vi "Main 2.vi"() -> ()   [LabVIEW 2016, in "MyHostCode.lvlib"]
doc: "This VI was generated automatically using the FPGA Wizard. You can modify the VI normally."
uses:
  MyHostCode.lvlib
  FPGACode/Lead Enum.ctl
  Trigger Params.ctl
  FPGACode/Channel Enum.ctl
  <vilib>/Utility/file.llb/Write To Spreadsheet File (I64).vi
  <vilib>/FPGAPlugInAG/USB-7856R OEM/niLvFpga_Open_USB-7856R OEM.vi
  <vilib>/rvi/interface/common/dynamic/niFpgaDynamicAddResources.vi
  <vilib>/FPGAPlugInAG/Dynamic/niLvFpga_Reset_Dynamic.vi
  <vilib>/FPGAPlugInAG/Dynamic/niLvFpga_Run_Dynamic.vi
  <vilib>/Utility/error.llb/Error Cluster From Error Code.vi
  <vilib>/rvi/errors/niLvFpgaAdjustHostInterfaceError.vi
  <vilib>/FPGAPlugInAG/Dynamic/niLvFpga_Close_Dynamic.vi
  <vilib>/rvi/interface/nirviOpenFPGA/nirviOpenFPGA.xnode
  FPGA Bitfiles/ECGPWMAdaptiveFi_FPGATarget3_ECGAFSPIInput2_KN+BrzZOq5c.lvbitx
  <vilib>/rvi/interface/nirviMethod/nirviMethod.xnode
  <vilib>/rvi/interface/nirviReadWriteControl/nirviReadWriteControl.xnode
  <vilib>/rvi/interface/nirviCloseFPGA/nirviCloseFPGA.xnode
  <vilib>/rvi/interface/Simulation/niFpgaSimulationCallBeginRW.vi
  <vilib>/FPGAPlugInAG/Dynamic/niLvFpga_ReadFifo_Dynamic.vi
  <vilib>/rvi/errors/niLvFpgaMergeErrorWithErrorCode.vi
  NiFpgaLv.dll
panel:
  in  "Path":path=path "C:/Users/IFEUser/Documents/LabVIEW Data/Saved Data/test.txt"
  in  "Record":bool
  in  "Beta":u8(slide)=1 scale=0.0..3.0
  in  "Sensis\nECG Scaling":i16=1 caption="ECG Output\nScaling" min=1 max=100 step=1
  in  "Tab Control":enum32{"Main", "Utilities"}(tab)
  in  "IBP2":T1={"Scale"=0.169921875, "Offset"=-1935.0} {"Scale" format="%#_3g"}
  out "ECG":i16[][](graph)
  out "Invasive Blood Pressure":i16[][](graph)=[[-20, 4166], [-20, 4166], [-20, 4165], [-20, 4165], [-19, 4165], [-19, 4165], [-18, 4163], [-18, 4165], [-18, 4166], [-18, 4166], [-18, 4166], [-18, 4165], [-18, 4165], [-18, 4164], [-18, 4164], [-18, 4165], [-19, 4166], [-20, 4166], [-20, 4164], [-20, 4164], [-20, 4165], [-20, 4165], [-19, 4165], [-19, 4164], [-18, 4165], [-18, 4166], [-18, 4165], [-18, 4166], [-18, 4165], [-18, 4165], [-18, 4165], [-18, 4165], [-19, 4165], [-20, 4165], [-20, 4165], [-20, 4165], [-20, 4166], [-20, 4167], [-20, 4166], [-19, 4164], [-18, 4163], [-18, 4164], [-18, 4165], [-18, 4166], [-17, 4165], [-18, 4166], [-18, 4166], [-18, 4165], [-18, 4166], [-19, 4165], [-20, 4164], [-20, 4165], [-20, 4166], [-20, 4166], [-20, 4167]]
  in  "Trigger 2":T2={"Channel"=enum."II", "Threshold"=1000, "d/dt"=FALSE, "Invert"=FALSE}
  out "Trigger":i16[][](graph)
  in  "IBP Filter":bool
  in  "Plot Info":T5={"Element"={"Lead"=enum."I", "Filter"=TRUE}, "Element 2"={"Lead"=enum."II", "Filter"=TRUE}, "Element 3"={"Lead"=enum."III", "Filter"=TRUE}}
  in  "IBP1":T1={"Scale"=0.1669921875, "Offset"=-1795.0} {"Scale" format="%#_4g"}
  in  "Invert IBP PWM":bool=TRUE
  in  "Invert ECG PWM":bool=TRUE
  out "Gradients":i16[][](graph)
  in  "Offset":cluster{"X":i16, "Y":i16, "Z":i16} {"Z" format="%.2f"; "Y" format="%.2f"; "X" format="%.2f"}
  in  "High Pass Filter":bool
  out "Taps":dbl[](graph)
  out "Weights":dbl[](graph)
  out "Beta Product":fxp<+/-,32,-1> format="%.3e"
  out "Weighted Sum":fxp<+/-,33,19> format="%.3e"
  in  "Channel":i32
  in  "ECG Input\nGain":u16(ring)=1 items=["1"=1, "2"=2, "3"=3, "4"=4, "6"=0, "8"=5, "12"=6]
  in  "ECG Beta":fxp<+/-,32,-16>=1.000088900582341e-11 format="%.3e"
  in  "Filter Size":i16=100
  in  "IBP Beta":fxp<+/-,32,-16> format="%.3e"
  out "Loop Time":u32
  in  "Reset":bool
  out "Actual Loop Rate (Ticks)":u32
  out "Late? Latched":bool
  in  "Start":bool
  in  "Loop Rate (Hz)":dbl=10000.0
  out "Calculated Rate (Hz)":dbl
  out "error out":errorcluster
  in  "Global Stop":bool
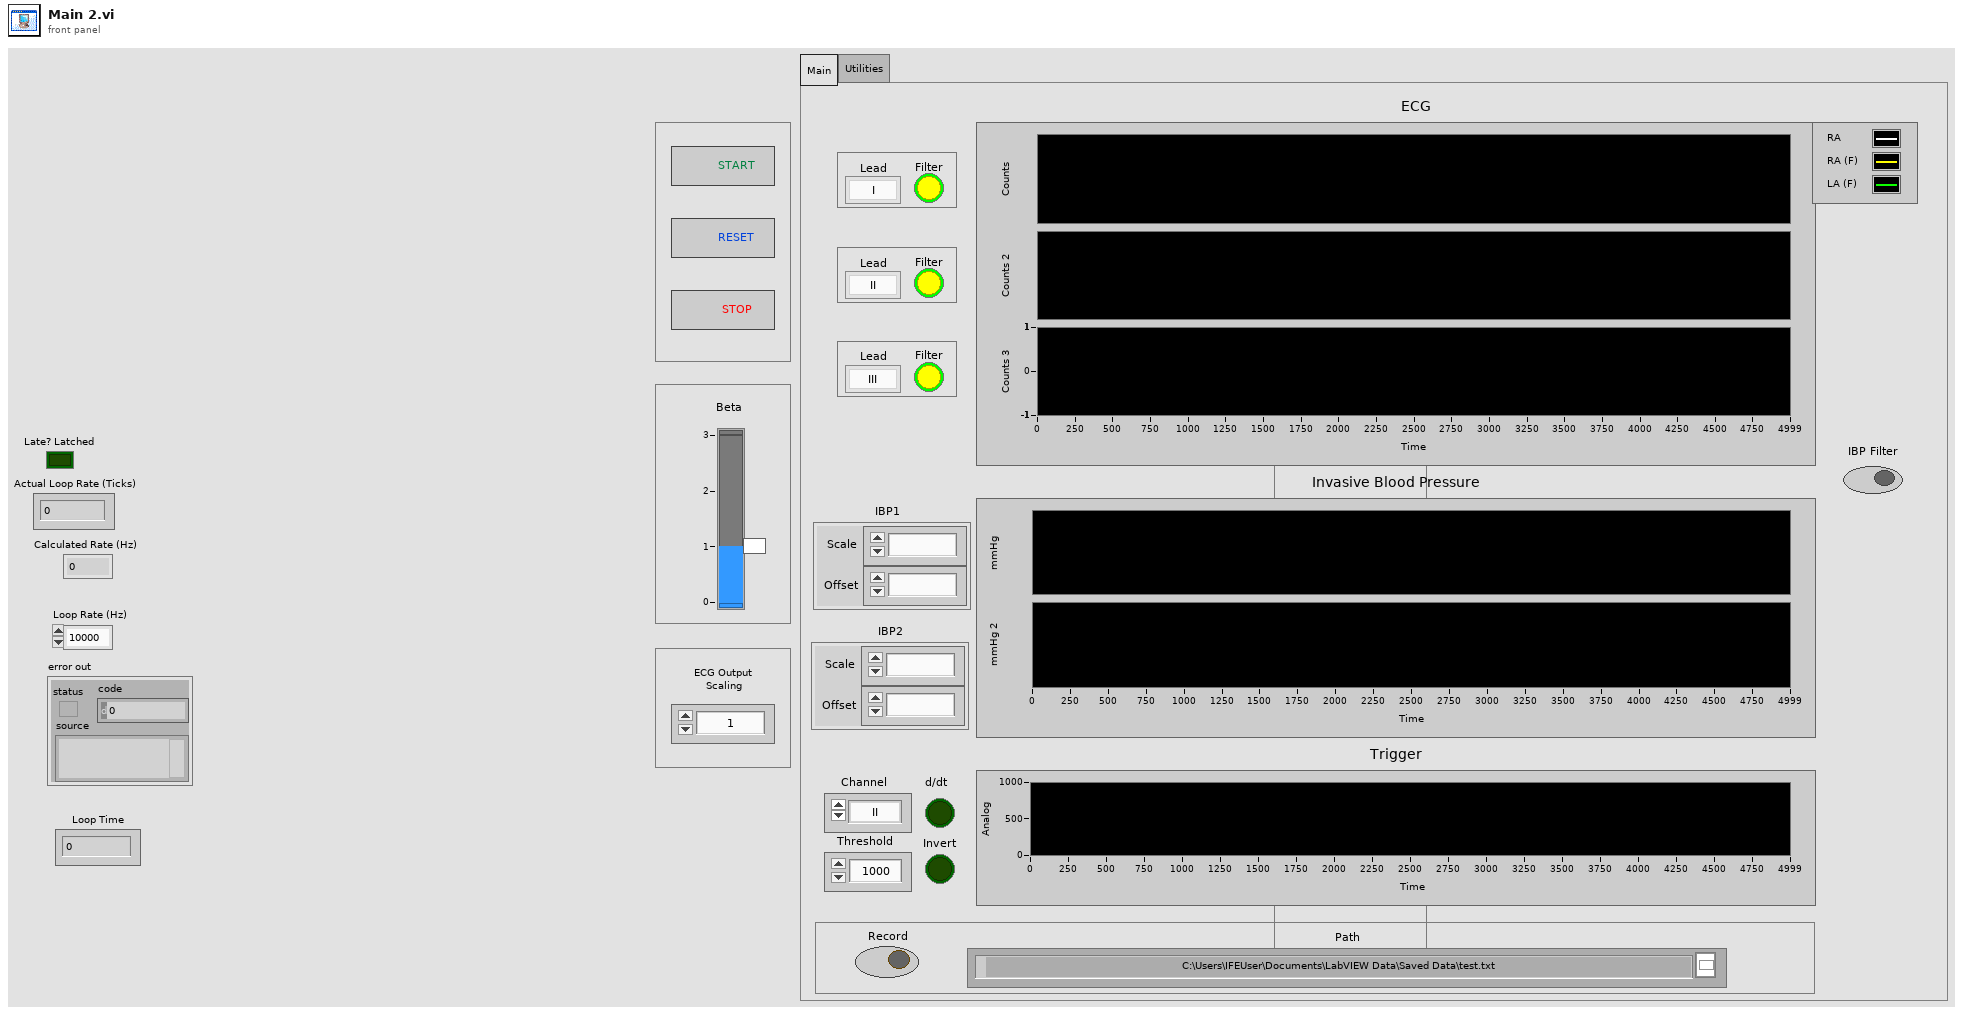
[diagram p1: front panel]
types:
  T1 = cluster{"Scale":fxp<+/-,16,5>, "Offset":fxp<+/-,16,16>}
  T2 = typedef "Trigger Params.ctl" = cluster{"Channel":T3, "Threshold":i16, "d/dt":bool, "Invert":bool}
  T3 = typedef "Channel Enum.ctl" = enum16{"RA", "LA", "LL", "V1", "V2", "V3", "V4", "V5", "V6", "I", "II", "III", "aVR", "aVL", "aVF", "Vw", "IBP1", "IBP2"}
  T4 = typedef "Lead Enum.ctl" = enum16{"RA", "LA", "LL", "V1", "V2", "V3", "V4", "V5", "V6", "I", "II", "III", "aVR", "aVL", "aVF", "Vw"}
  T5 = cluster{"Element":cluster{"Lead":T4, "Filter":bool}, "Element 2":cluster{"Lead":T4, "Filter":bool}, "Element 3":cluster{"Lead":T4, "Filter":bool}}
  T6 = enum8{"Enabled", "Disabled", "Disabled and Grayed Out"}
  T7 = typedef "LVOffsetAndMultiplierTypeDef.ctl" = cluster{"Offset":dbl, "Multiplier":dbl}
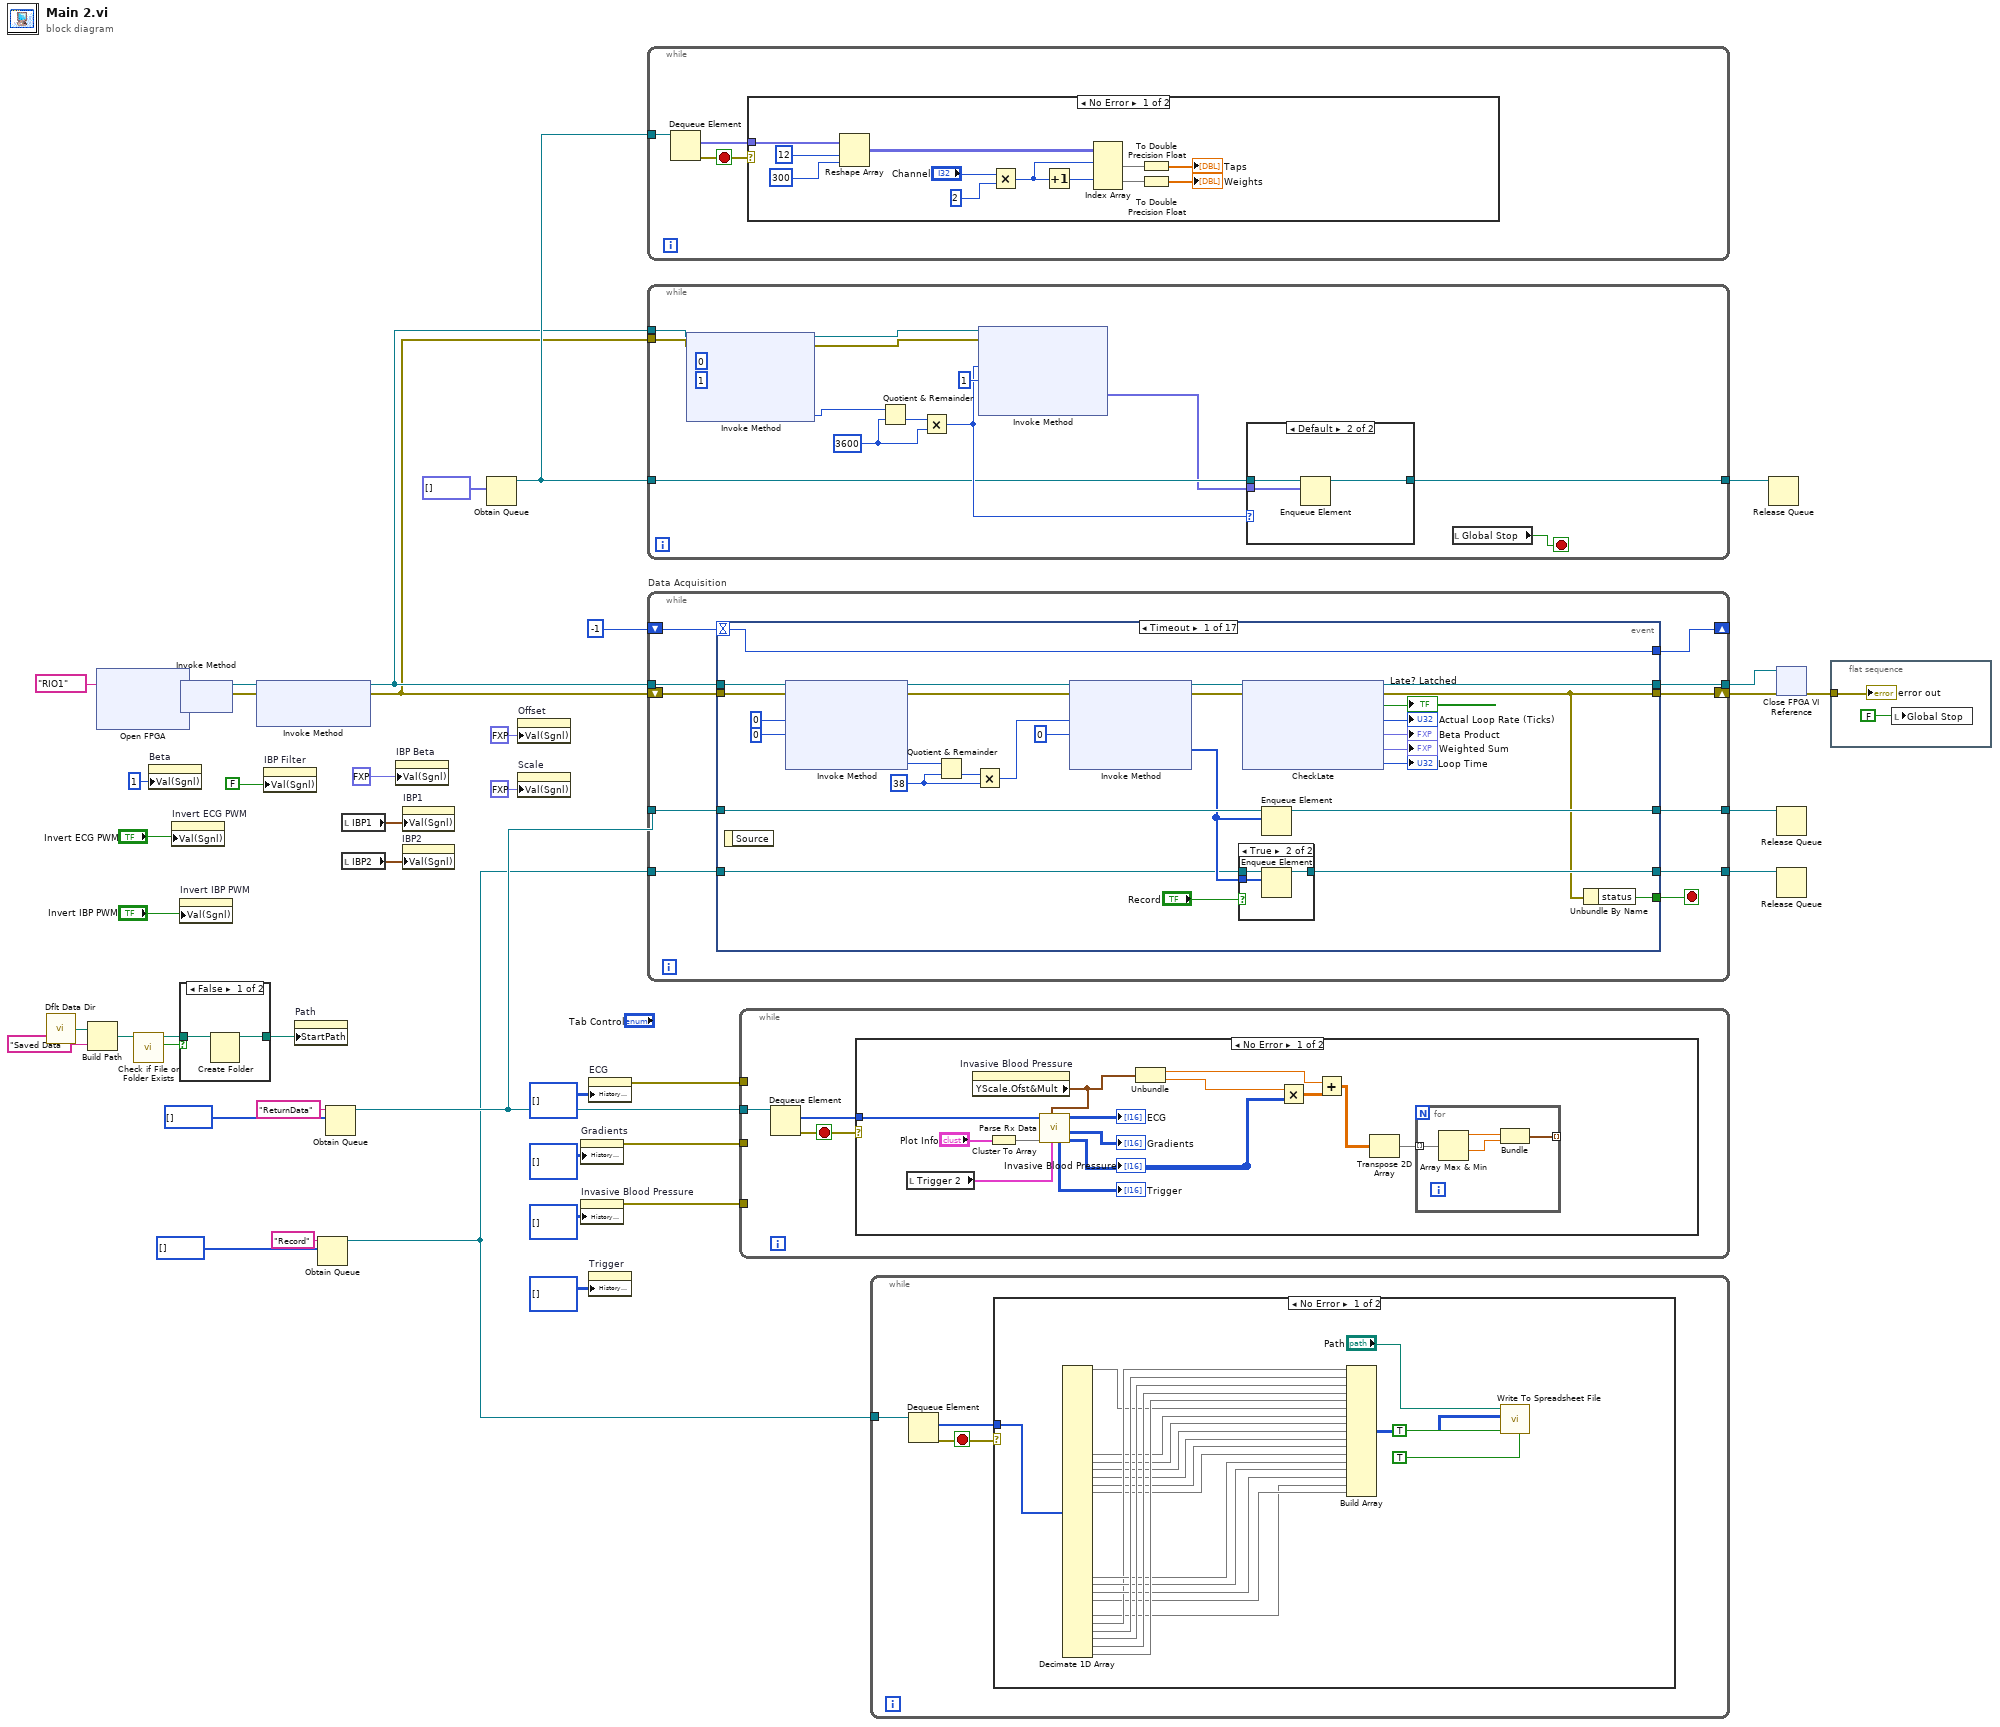
[diagram p0: block diagram]
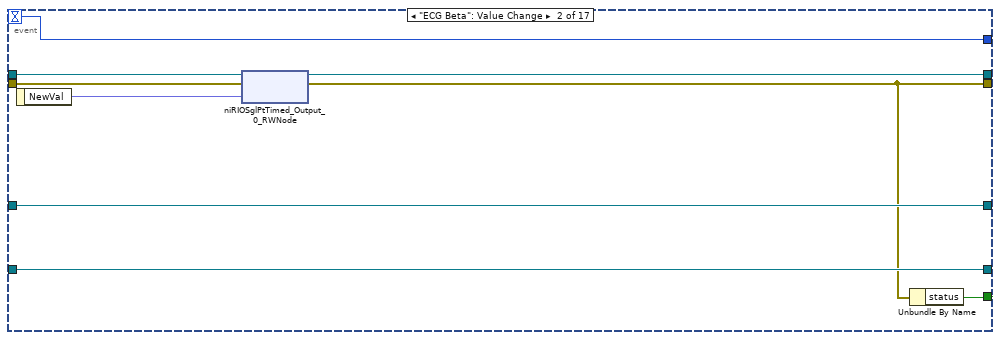
[diagram p4: hidden frame]
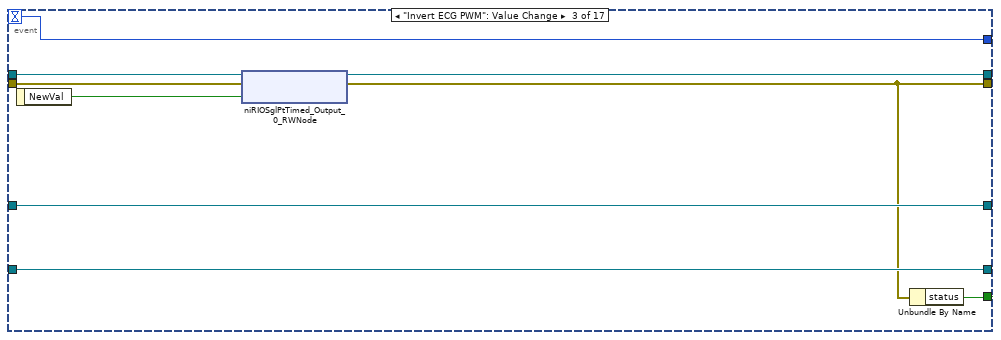
[diagram p5: hidden frame]
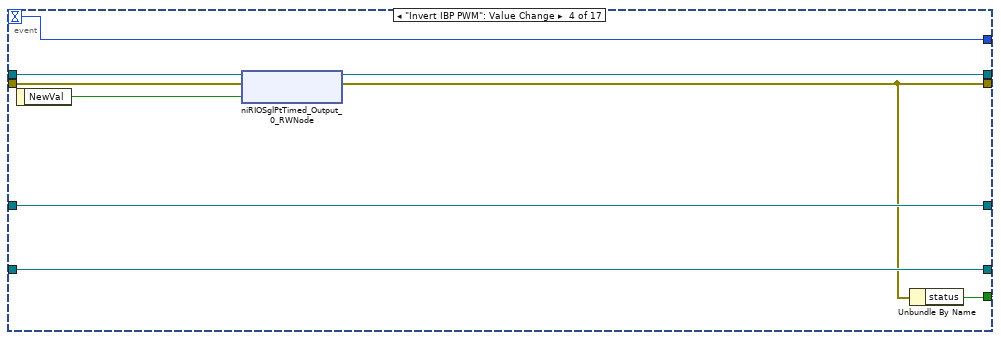
[diagram p6: hidden frame]
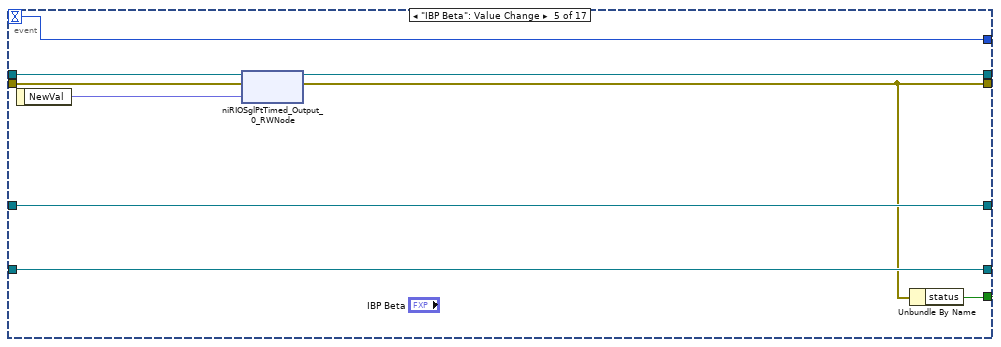
[diagram p7: hidden frame]
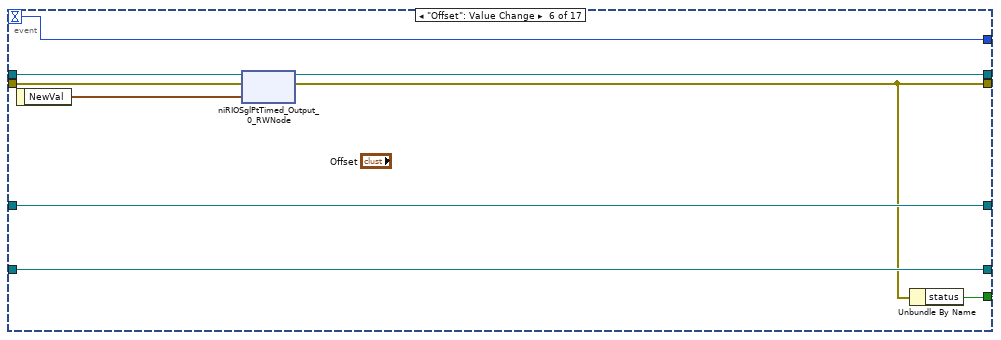
[diagram p8: hidden frame]
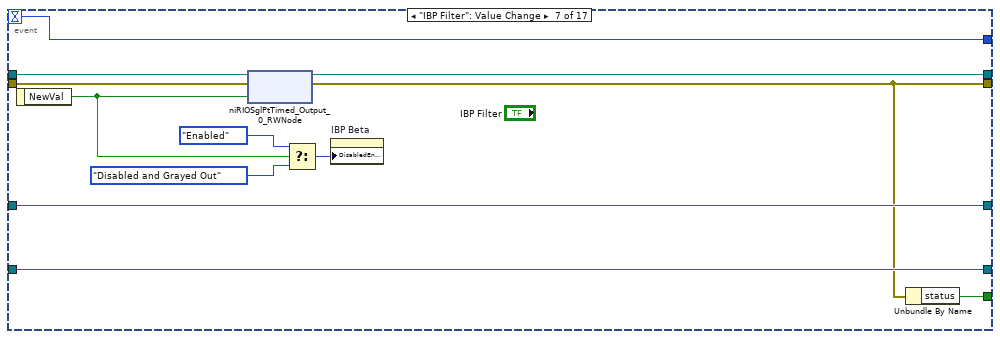
[diagram p9: hidden frame]
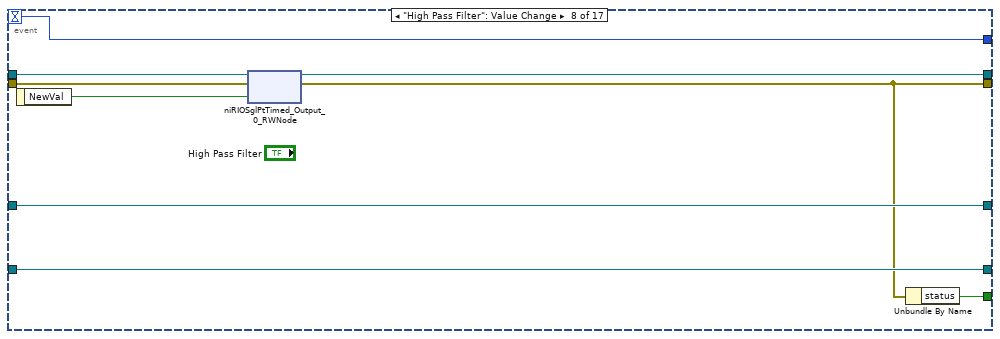
[diagram p10: hidden frame]
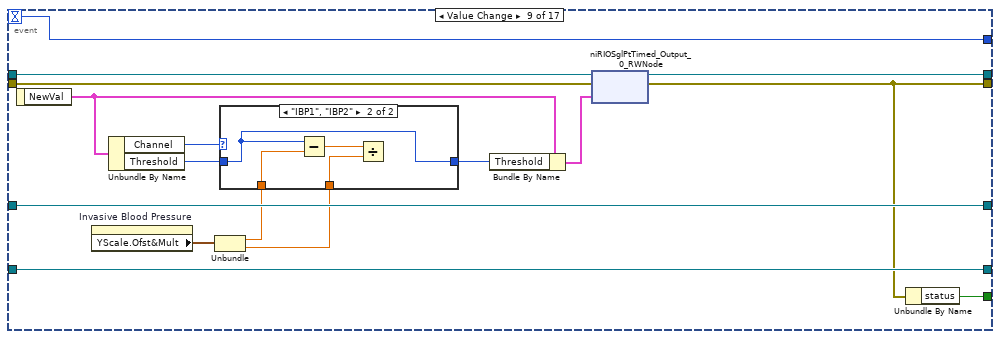
[diagram p11: hidden frame]
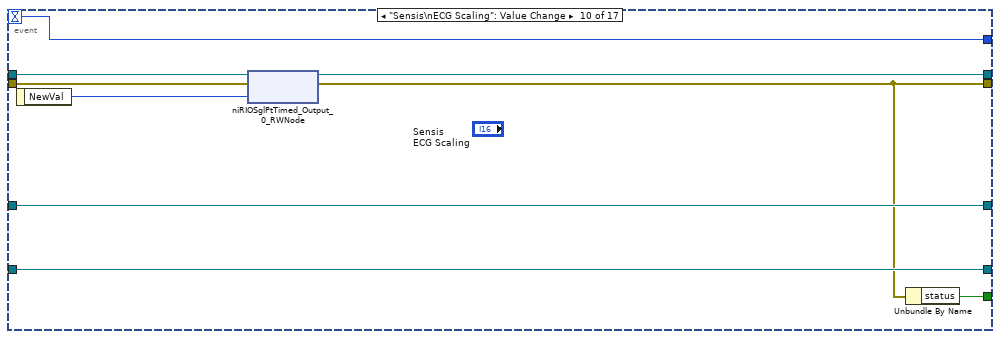
[diagram p13: hidden frame]
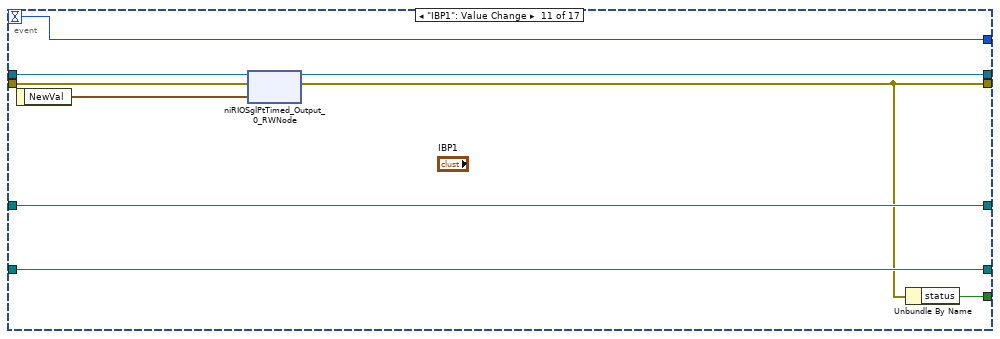
[diagram p14: hidden frame]
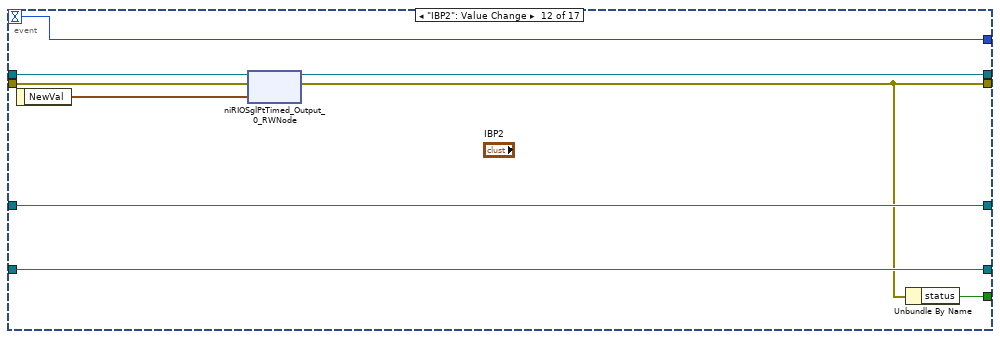
[diagram p15: hidden frame]
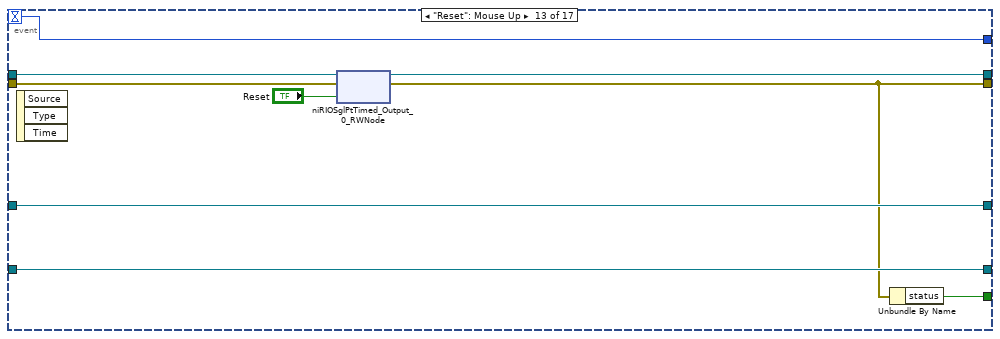
[diagram p16: hidden frame]
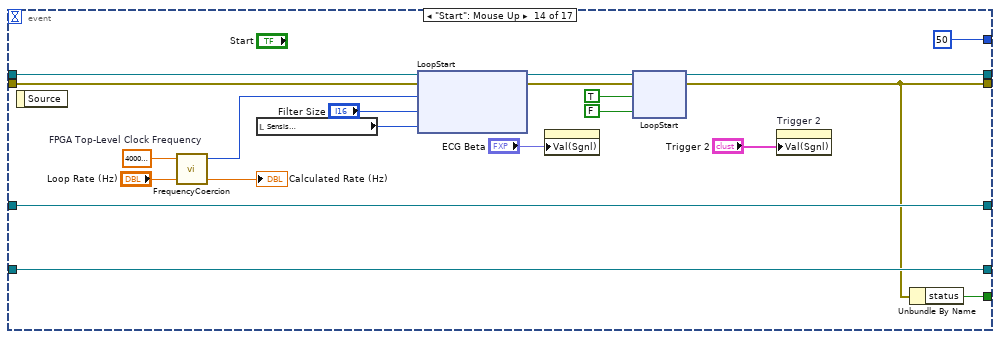
[diagram p17: hidden frame]
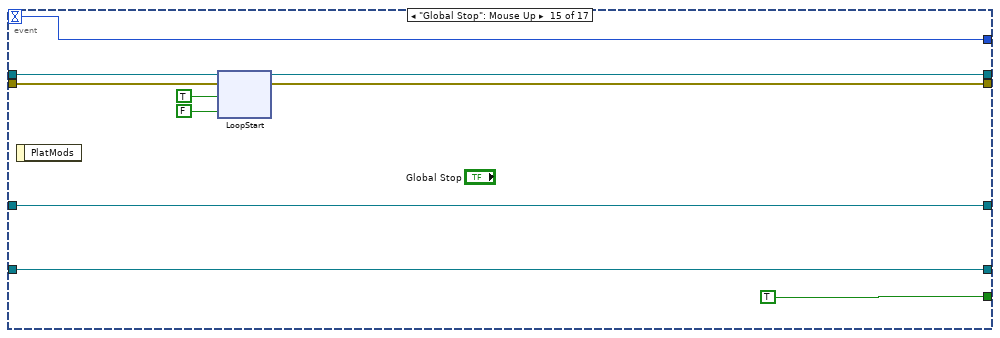
[diagram p18: hidden frame]
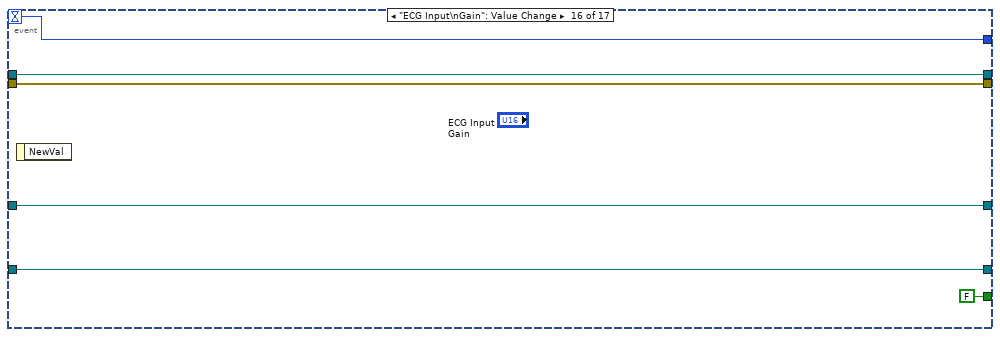
[diagram p19: hidden frame]
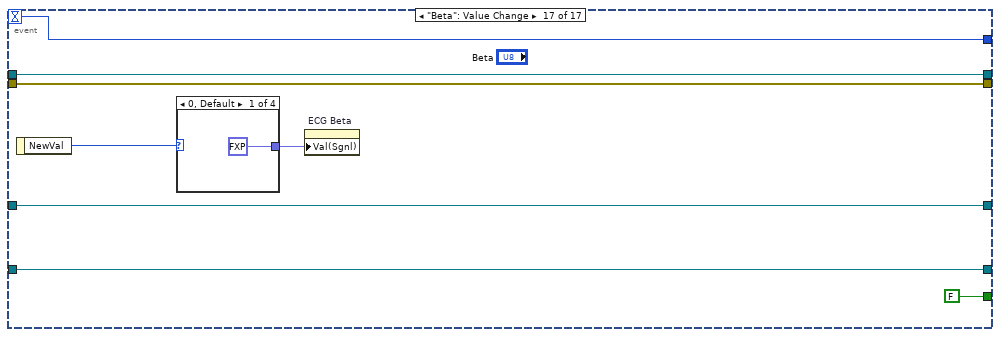
[diagram p20: hidden frame]
diagram:
  n1 = call <vilib>:"Dflt Data Dir.vi"() -> ("App:Default Data Directory"=w10:path)
  n2 = Build Path(base path=w10, name or relative path="Saved Data") -> (appended path=w8:path)
  n3 = xnode ("Open FPGA")("resource name"=tag "RIO1") -> ("FPGA VI Reference Out"=w43:refnum<k20>, "error out"=w42:errorcluster)  [unwired: 1 in]
  n4 = call <vilib>:"Check if File or Folder Exists.vi"("path"=w8) -> ("file or folder exists?"=w7:bool, "dup path"=w6:path)  [unwired: 8 in, 1 out]
  n5 = property on="Beta" class="Slide (strict)"("Val(Sgnl)"=u8 1 ("Value (Signaling)")) -> ()  [unwired: 2 in, 2 out]
  n6 = property on="Invert ECG PWM" class="Bool (strict)"("Val(Sgnl)"="Invert ECG PWM") -> ()  [unwired: 2 in, 2 out]
  n7 = property on="Invert IBP PWM" class="Bool (strict)"("Val(Sgnl)"="Invert IBP PWM") -> ()  [unwired: 2 in, 2 out]
  n8 = case shown="False" w7 {
    tunnel: w6 -> [w46 w47]
    tunnel: [w45 w47] -> w5
    frame False {
      n9 = Create Folder(path (use dialog)=w46) -> (created path=w45:path)  [unwired: 2 in, 2 out]
    }
    frame True {
    }
  }
  n10 = xnode ("Invoke Method")("FPGA VI Reference In"=w43, "error in"=w42) -> ("FPGA VI Reference Out"=w20:refnum<k20>, "error out"=w44:errorcluster)
  n11 = xnode ("Invoke Method")("FPGA VI Reference In"=w20, "error in"=w44) -> ("FPGA VI Reference Out"=w18:refnum<k20>, "error out"=w17:errorcluster)  [unwired: 1 in]
  n12 = property on="IBP Filter" class="Bool (strict)"("Val(Sgnl)"=FALSE ("Value (Signaling)")) -> ()  [unwired: 2 in, 2 out]
  n13 = property on="Path" class="Path"("StartPath"=w5) -> ()  [unwired: 2 in, 2 out]
  n14 = Obtain Queue(name (unnamed)="Record", element data type=i16[] []) -> (queue out=w28:refnum<queue>)  [unwired: 3 in, 2 out]
  n15 = Obtain Queue(name (unnamed)="ReturnData", element data type=i16[] []) -> (queue out=w36:refnum<queue>)  [unwired: 3 in, 2 out]
  n16 = local read "IBP1"() -> (w4:T1)
  n17 = local read "IBP2"() -> (w3:T1)
  n18 = property on="IBP Beta" class="DigNum (strict)"("Val(Sgnl)"=fxp<+/-,32,-16> 0.0 ("Value (Signaling)")) -> ()  [unwired: 2 in, 2 out]
  n19 = property on="IBP1" class="Clust (strict)"("Val(Sgnl)"=w4) -> ()  [unwired: 2 in, 2 out]
  n20 = property on="IBP2" class="Clust (strict)"("Val(Sgnl)"=w3) -> ()  [unwired: 2 in, 2 out]
  n21 = Obtain Queue(element data type=fxp<+/-,32,16>[] [] ("Data")) -> (queue out=w23:refnum<queue>)  [unwired: 4 in, 2 out]
  n22 = property on="Offset" class="DigNum (strict)"("Val(Sgnl)"=fxp<+/-,16,16> 0.0 ("Value (Signaling)")) -> ()  [unwired: 2 in, 2 out]
  n23 = property on="Scale" class="DigNum (strict)"("Val(Sgnl)"=fxp<+/-,16,5> 1.0 ("Value (Signaling)")) -> ()  [unwired: 2 in, 2 out]
  n24 = property on="Gradients" class="WFChart (strict)"("History Data"=i16[][] []) -> (error out=w33:errorcluster)  [unwired: 2 in, 1 out]
  n25 = property on="Invasive Blood Pressure" class="WFChart (strict)"("History Data"=i16[][] []) -> (error out=w25:errorcluster)  [unwired: 2 in, 1 out]
  n26 = property on="ECG" class="WFChart (strict)"("History Data"=i16[][] []) -> (error out=w34:errorcluster)  [unwired: 2 in, 1 out]
  n27 = property on="Trigger" class="WFChart (strict)"("History Data"=i16[][] []) -> ()  [unwired: 2 in, 2 out]
  n28 = while {
    tunnel: w23 -> [w50]
    stop <- w48 stop-if-true
    n29 = Dequeue Element(queue=w50) -> (element=w49:fxp<+/-,32,16>[], error out=w48:errorcluster)  [unwired: 2 in, 2 out]
    n30 = case shown="No Error" w48 {
      tunnel: w49 -> [w62 _]
      frame No Error {
        n31 = Reshape Array(w62, 12 ("dimension size"), 300 ("dimension size")) -> (w58:fxp<+/-,32,16>[][])
        n32 = Multiply(x="Channel", y=2) -> (x*y=w51:i32)
        n33 = Increment(x=w51) -> (x+1=w52:i32)
        n34 = Index Array(array=w58, index (row) #1=w51, index (row) #2=w52) -> (element #1=w57:fxp<+/-,32,16>[], element #2=w56:fxp<+/-,32,16>[])  [unwired: 2 in]
        n35 = To Double Precision Float(number=w57) -> (double precision float=→"Taps":dbl[])
        n36 = To Double Precision Float(number=w56) -> (double precision float=→"Weights":dbl[])
      }
      frame Error {
      }
    }
  }
  n37 = while {
    tunnel: w18 -> [w77]
    tunnel: w17 -> [w76]
    tunnel: w23 -> [w65]
    tunnel: [w63] -> w22
    stop <- w68 stop-if-true
    w70 = u32 3600 ("y")
    n38 = xnode "Invoke Method"("FPGA VI Reference In"=w77, "error in"=w76, "Number of Elements"=u32 0, "Timeout (ms)"=1) -> ("FPGA VI Reference Out"=w73:refnum<k20>, "error out"=w72:errorcluster, "Elements Remaining"=w69:u32)  [unwired: 1 out]
    n39 = Quotient & Remainder(x=w69, y=w70) -> (floor(x/y)=w71:u32)  [unwired: 1 out]
    n40 = Multiply(x=w71, y=w70) -> (x*y=w66:u32)
    n41 = xnode "Invoke Method"("FPGA VI Reference In"=w73, "error in"=w72, "Number of Elements"=w66, "Timeout (ms)"=1) -> ("Data"=w64:fxp<+/-,32,16>[])  [unwired: 3 out]
    n42 = case shown="Default" w66 {
      tunnel: w65 -> [w78 w81]
      tunnel: w64 -> [_ w80]
      tunnel: [w78 w79] -> w63
      frame 0 {
      }
      frame Default {
        n43 = Enqueue Element(queue=w81, element=w80) -> (queue out=w79:refnum<queue>)  [unwired: 2 in, 2 out]
      }
    }
    n44 = local read "Global Stop"() -> (w68:bool)
  }
  n45 = while "Data Acquisition" {
    tunnel: w18 -> [w88]
    shift-right: [w92] -> w41
    shift-left: w17 -> [w89]
    tunnel: [w90] -> w39
    tunnel: w36 -> [w87]
    tunnel: [w86] -> w31
    tunnel: w28 -> [w85]
    tunnel: [w84] -> w27
    shift-right: [w82] -> _
    shift-left: -1 -> [w83]
    stop <- w91 stop-if-true
    n46 = event shown="[0] Timeout" {
      selector: _ -> [_ _ _ _ _ _ _ _ _ _ _ _ _ _ _ _ _]
      dyn-events: _ -> [_ _ _ _ _ _ _ _ _ _ _ _ _ _ _ _ _]
      timeout: w83 -> [w95 w127 w136 w145 w154 w163 w176 w184 w201 w215 w224 w233 w241 _ w270 w281 w290]
      tunnel: [w94 w126 w135 w144 w153 w162 w175 w183 w200 w214 w223 w232 w240 w251 w271 w282 w289] -> w92
      tunnel: [w93 w125 w134 w143 w152 w161 w174 w182 w199 w213 w222 w231 w239 w250 TRUE FALSE ("status") FALSE ("status")] -> w91
      tunnel: [w120 w131 w140 w149 w158 w167 w179 w188 w204 w218 w227 w236 w245 w255 w272 w283 w291] -> w90
      tunnel: w89 -> [w97 w132 w141 w150 w159 w168 w180 w189 w205 w219 w228 w237 w246 w265 w273 w282 w289]
      tunnel: w88 -> [w98 w133 w142 w151 w160 w169 w181 w190 w206 w220 w229 w238 w247 w266 w274 w283 w291]
      tunnel: w87 -> [w109 w129 w138 w147 w156 w165 w178 w186 w203 w217 w226 w235 w244 w264 w277 w280 w288]
      tunnel: [w105 w129 w138 w147 w156 w165 w178 w186 w203 w217 w226 w235 w244 w264 w277 w280 w288] -> w86
      tunnel: w85 -> [w102 w128 w137 w146 w155 w164 w177 w185 w202 w216 w225 w234 w243 w263 w276 w279 w287]
      tunnel: [w96 w128 w137 w146 w155 w164 w177 w185 w202 w216 w225 w234 w243 w263 w276 w279 w287] -> w84
      tunnel: [w95 w127 w136 w145 w154 w163 w176 w184 w201 w215 w224 w233 w241 50 w270 w281 w290] -> w82
      event Timeout {
        w107 = u32 38 ("y")
        n47 = event-data() -> ()  [unwired: 1 in, 1 out]
        n48 = xnode "Invoke Method"("FPGA VI Reference In"=w98, "error in"=w97, "Number of Elements"=u32 0, "Timeout (ms)"=0) -> ("FPGA VI Reference Out"=w115:refnum<k20>, "error out"=w114:errorcluster, "Elements Remaining"=w113:u32)  [unwired: 1 out]
        n49 = Quotient & Remainder(x=w113, y=w107) -> (floor(x/y)=w108:u32)  [unwired: 1 out]
        n50 = Multiply(x=w108, y=w107) -> (x*y=w106:u32)
        n51 = xnode "Invoke Method"("FPGA VI Reference In"=w115, "error in"=w114, "Number of Elements"=w106, "Timeout (ms)"=0) -> ("FPGA VI Reference Out"=w111:refnum<k20>, "error out"=w110:errorcluster, "Data"=w103:i16[])  [unwired: 1 out]
        n52 = case shown="True" "Record" {
          tunnel: w103 -> [_ w124]
          tunnel: w102 -> [w121 w123]
          tunnel: [w121 w122] -> w96
          frame False {
          }
          frame True {
            n53 = Enqueue Element(queue=w123, element=w124) -> (queue out=w122:refnum<queue>)  [unwired: 2 in, 2 out]
          }
        }
        n54 = xnode ("CheckLate")("FPGA VI Reference In"=w111, "error in"=w110) -> ("FPGA VI Reference Out"=w120:refnum<k20>, "error out"=w94:errorcluster, "Late? Latched"=→"Late? Latched":bool, "Actual Loop Rate (Ticks)"=→"Actual Loop Rate (Ticks)":u32, "BetaProduct"=→"Beta Product":fxp<+/-,32,-1>, "WeightSum"=→"Weighted Sum":fxp<+/-,33,19>, "Loop Time"=→"Loop Time":u32)
        n55 = Enqueue Element(queue=w109, element=w103) -> (queue out=w105:refnum<queue>)  [unwired: 2 in, 2 out]
        n56 = Unbundle By Name(w94) -> ("status"=w93:bool)
      }
      event "ECG Beta": Value Change {
        n57 = event-data() -> ("NewVal"=w130:fxp<+/-,32,-16>)  [unwired: 1 in]
        n58 = xnode ("niRIOSglPtTimed_Output_0_RWNode")("FPGA VI Reference In"=w133, "error in"=w132, "Beta ECG"=w130) -> ("FPGA VI Reference Out"=w131:refnum<k20>, "error out"=w126:errorcluster)
        n59 = Unbundle By Name(w126) -> ("status"=w125:bool)
      }
      event "Invert ECG PWM": Value Change {
        n60 = event-data() -> ("NewVal"=w139:bool)  [unwired: 1 in]
        n61 = xnode ("niRIOSglPtTimed_Output_0_RWNode")("FPGA VI Reference In"=w142, "error in"=w141, "Invert PWM ECG"=w139) -> ("FPGA VI Reference Out"=w140:refnum<k20>, "error out"=w135:errorcluster)
        n62 = Unbundle By Name(w135) -> ("status"=w134:bool)
      }
      event "Invert IBP PWM": Value Change {
        n63 = event-data() -> ("NewVal"=w148:bool)  [unwired: 1 in]
        n64 = xnode ("niRIOSglPtTimed_Output_0_RWNode")("FPGA VI Reference In"=w151, "error in"=w150, "Invert PWM IBP"=w148) -> ("FPGA VI Reference Out"=w149:refnum<k20>, "error out"=w144:errorcluster)
        n65 = Unbundle By Name(w144) -> ("status"=w143:bool)
      }
      event "IBP Beta": Value Change {
        n66 = event-data() -> ("NewVal"=w157:fxp<+/-,32,-16>)  [unwired: 1 in]
        n67 = xnode ("niRIOSglPtTimed_Output_0_RWNode")("FPGA VI Reference In"=w160, "error in"=w159, "Beta IBP"=w157) -> ("FPGA VI Reference Out"=w158:refnum<k20>, "error out"=w153:errorcluster)
        n68 = Unbundle By Name(w153) -> ("status"=w152:bool)
      }
      event "Offset": Value Change {
        n69 = event-data() -> ("NewVal"=w166:cluster{"X":i16, "Y":i16, "Z":i16})  [unwired: 1 in]
        n70 = xnode ("niRIOSglPtTimed_Output_0_RWNode")("FPGA VI Reference In"=w169, "error in"=w168, "Offset"=w166) -> ("FPGA VI Reference Out"=w167:refnum<k20>, "error out"=w162:errorcluster)
        n71 = Unbundle By Name(w162) -> ("status"=w161:bool)
      }
      event "IBP Filter": Value Change {
        n72 = event-data() -> ("NewVal"=w173:bool)  [unwired: 1 in]
        n73 = xnode ("niRIOSglPtTimed_Output_0_RWNode")("FPGA VI Reference In"=w181, "error in"=w180, "IBP Filter"=w173) -> ("FPGA VI Reference Out"=w179:refnum<k20>, "error out"=w175:errorcluster)
        n74 = Select(t=T6."Enabled" ("Disabled"), s=w173, f=T6."Disabled and Grayed Out" ("Disabled")) -> (s? t:f=w170:T6)
        n75 = property on="IBP Beta" class="DigNum (strict)"("DisabledEnum"=w170) -> ()  [unwired: 2 in, 2 out]
        n76 = Unbundle By Name(w175) -> ("status"=w174:bool)
      }
      event "High Pass Filter": Value Change {
        n77 = event-data() -> ("NewVal"=w187:bool)  [unwired: 1 in]
        n78 = xnode ("niRIOSglPtTimed_Output_0_RWNode")("FPGA VI Reference In"=w190, "error in"=w189, "HPF"=w187) -> ("FPGA VI Reference Out"=w188:refnum<k20>, "error out"=w183:errorcluster)
        n79 = Unbundle By Name(w183) -> ("status"=w182:bool)
      }
      event Value Change {
        n80 = event-data() -> ("NewVal"=w196:T2)  [unwired: 1 in]
        n81 = property on="Invasive Blood Pressure" class="WFChart (strict)"() -> ("YScale.Ofst&Mult"=w193:T7)  [unwired: 2 in, 2 out]
        n82 = Unbundle By Name(w196) -> ("Channel"=w198:T3, "Threshold"=w197:i16)
        n83 = Unbundle(w193) -> ("Offset"=w192:dbl, "Multiplier"=w191:dbl)
        n84 = case shown="\"IBP1\", \"IBP2\"" w198 {
          tunnel: w197 -> [w207 w208]
          tunnel: [w207 w208] -> w195
          tunnel: w192 -> [_ w211]
          tunnel: w191 -> [_ w209]
          frame Default {
          }
          frame "IBP1", "IBP2" {
            n85 = Subtract(x=w208, y=w211) -> (x-y=w210:dbl)
            n86 = Divide(x=w210, y=w209) -> ()  [unwired: 1 out]
          }
        }
        n87 = Bundle By Name(cluster=w196, "Threshold"=w195) -> (w194:T2)
        n88 = xnode ("niRIOSglPtTimed_Output_0_RWNode")("FPGA VI Reference In"=w206, "error in"=w205, "Trigger"=w194) -> ("FPGA VI Reference Out"=w204:refnum<k20>, "error out"=w200:errorcluster)
        n89 = Unbundle By Name(w200) -> ("status"=w199:bool)
      }
      event "Sensis\nECG Scaling": Value Change {
        n90 = event-data() -> ("NewVal"=w212:i16)  [unwired: 1 in]
        n91 = xnode ("niRIOSglPtTimed_Output_0_RWNode")("FPGA VI Reference In"=w220, "error in"=w219, "ECG Scale"=w212) -> ("FPGA VI Reference Out"=w218:refnum<k20>, "error out"=w214:errorcluster)
        n92 = Unbundle By Name(w214) -> ("status"=w213:bool)
      }
      event "IBP1": Value Change {
        n93 = event-data() -> ("NewVal"=w221:T1)  [unwired: 1 in]
        n94 = xnode ("niRIOSglPtTimed_Output_0_RWNode")("FPGA VI Reference In"=w229, "error in"=w228, "IBP1"=w221) -> ("FPGA VI Reference Out"=w227:refnum<k20>, "error out"=w223:errorcluster)
        n95 = Unbundle By Name(w223) -> ("status"=w222:bool)
      }
      event "IBP2": Value Change {
        n96 = event-data() -> ("NewVal"=w230:T1)  [unwired: 1 in]
        n97 = xnode ("niRIOSglPtTimed_Output_0_RWNode")("FPGA VI Reference In"=w238, "error in"=w237, "IBP1 2"=w230) -> ("FPGA VI Reference Out"=w236:refnum<k20>, "error out"=w232:errorcluster)
        n98 = Unbundle By Name(w232) -> ("status"=w231:bool)
      }
      event "Reset": Mouse Up {
        n99 = event-data() -> ()  [unwired: 1 in, 3 out]
        n100 = xnode ("niRIOSglPtTimed_Output_0_RWNode")("FPGA VI Reference In"=w247, "error in"=w246, "Reset"="Reset") -> ("FPGA VI Reference Out"=w245:refnum<k20>, "error out"=w240:errorcluster)
        n101 = Unbundle By Name(w240) -> ("status"=w239:bool)
      }
      event "Start": Mouse Up {
        w262 = 40000000.0  # FPGA Top-Level Clock Frequency
        n102 = event-data() -> ()  [unwired: 1 in, 1 out]
        n103 = call "FrequencyCoercion.vi"("Loop Rate (Hz)"="Loop Rate (Hz)", "FPGA Top-Level Clock Frequency"=w262) -> ("Actual Rate (Hz)"=→"Calculated Rate (Hz)":dbl, "FPGA Ticks"=w259:u32)  [unwired: 2 in]
        n104 = local read "Sensis\nECG Scaling"() -> (w248:i16)
        n105 = xnode ("LoopStart")("FPGA VI Reference In"=w266, "error in"=w265, "Loop Rate (Ticks)"=w259, "Filter Size"="Filter Size", "ECG Scale"=w248) -> ("FPGA VI Reference Out"=w257:refnum<k20>, "error out"=w256:errorcluster)
        n106 = property on="ECG Beta" class="DigNum (strict)"("Val(Sgnl)"="ECG Beta") -> ()  [unwired: 2 in, 2 out]
        n107 = xnode ("LoopStart")("FPGA VI Reference In"=w257, "error in"=w256, "Start"=TRUE ("Start 0"), "Start"=FALSE ("Start 0")) -> ("FPGA VI Reference Out"=w255:refnum<k20>, "error out"=w251:errorcluster)
        n108 = property on="Trigger 2" class="Clust (strict)"("Val(Sgnl)"="Trigger 2") -> ()  [unwired: 2 in, 2 out]
        n109 = Unbundle By Name(w251) -> ("status"=w250:bool)
      }
      event "Global Stop": Mouse Up {
        n110 = event-data() -> ()  [unwired: 1 in, 1 out]
        n111 = xnode ("LoopStart")("FPGA VI Reference In"=w274, "error in"=w273, "Stop"=TRUE ("stop"), "Stop"=FALSE ("stop")) -> ("FPGA VI Reference Out"=w272:refnum<k20>, "error out"=w271:errorcluster)
      }
      event "ECG Input\nGain": Value Change {
        n112 = event-data() -> ()  [unwired: 1 in, 1 out]
      }
      event "Beta": Value Change {
        n113 = event-data() -> ("NewVal"=w285:u8)  [unwired: 1 in]
        n114 = case shown="0, Default" w285 {
          tunnel: [fxp<+/-,32,-16> 0.0 ("Value (Signaling)") fxp<+/-,32,-16> 1.000088900582341e-11 ("Value (Signaling)") fxp<+/-,32,-16> 9.99982319171977e-11 ("Value (Signaling)") fxp<+/-,32,-16> 1.000000082740371e-09 ("Value (Signaling)")] -> w284
          frame 0, Default {
          }
          frame 1 {
          }
          frame 2 {
          }
          frame 3 {
          }
        }
        n115 = property on="ECG Beta" class="DigNum (strict)"("Val(Sgnl)"=w284) -> ()  [unwired: 2 in, 2 out]
      }
    }
  }
  n116 = while {
    tunnel: w36 -> [w298]
    tunnel: w34 -> [_]
    tunnel: w33 -> [_]
    tunnel: w25 -> [_]
    stop <- w297 stop-if-true
    n117 = Dequeue Element(queue=w298) -> (element=w296:i16[], error out=w297:errorcluster)  [unwired: 2 in, 2 out]
    n118 = case shown="No Error" w297 {
      tunnel: w296 -> [w312 _]
      frame No Error {
        n119 = local read "Trigger 2"() -> (w309:T2)
        n120 = property on="Invasive Blood Pressure" class="WFChart (strict)"() -> ("YScale.Ofst&Mult"=w299:T7)  [unwired: 2 in, 2 out]
        n121 = Cluster To Array(cluster="Plot Info") -> (array=w305:cluster{"Lead":T4, "Filter":bool}[])
        n122 = call "Parse Rx Data.vi"("Trigger"=w309, "Scale"=w299, "Plot Info"=w305, "Input Data"=w312) -> ("Pressures"=w301:i16[][], "Gradients"=→"Gradients":i16[][], "ECG Data"=→"ECG":i16[][], "Trigger"=→"Trigger":i16[][])  [unwired: 4 in]
        "Invasive Blood Pressure" <- w301
        n123 = Unbundle(w299) -> ("Offset"=w302:dbl, "Multiplier"=w304:dbl)
        n124 = Multiply(x=w304, y=w301) -> (x*y=w303:dbl[][])
        n125 = Add(x=w302, y=w303) -> (x+y=w300:dbl[][])
        n126 = Transpose 2D Array(2D array=w300) -> (transposed array=w306:dbl[][])
        n127 = for {
          tunnel: w306 -> [w316] mode=indexing
          tunnel: [w313] -> _ mode=indexing
          n128 = Array Max & Min(array=w316) -> (max value=w315:dbl, min value=w314:dbl)  [unwired: 2 out]
          n129 = Bundle(w315, w314) -> (w313:cluster{dbl, dbl})  [unwired: 1 in]
        }
      }
      frame Error {
      }
    }
  }
  n130 = while {
    tunnel: w28 -> [w317]
    stop <- w319 stop-if-true
    n131 = Dequeue Element(queue=w317) -> (element=w318:i16[], error out=w319:errorcluster)  [unwired: 2 in, 2 out]
    n132 = case shown="No Error" w319 {
      tunnel: w318 -> [w338 _]
      frame No Error {
        n133 = Decimate 1D Array(w338) -> (w321:i16[], w328:i16[], w327:i16[], w326:i16[], w325:i16[], w324:i16[], w320:i16[], w331:i16[], w332:i16[], w333:i16[], w323:i16[], w322:i16[], w329:i16[], w337:i16[], w336:i16[], w335:i16[], w334:i16[])  [unwired: 21 out]
        n134 = Build Array(w329, w337, w336, w335, w334, w321, w328, w327, w326, w325, w324, w320, w331, w332, w333, w322, w323) -> (w330:i16[][])
        n135 = call-poly <vilib>:"Write To Spreadsheet File.vi"("transpose? (no:F)"=TRUE, "append to file? (new file:F)"=TRUE, "2D data"=w330, "file path (dialog if empty)"="Path") -> ()  [unwired: 4 in, 1 out]
      }
      frame Error {
      }
    }
  }
  n136 = Release Queue(queue=w22) -> ()  [unwired: 2 in, 3 out]
  n137 = xnode ("Close FPGA VI Reference")("FPGA VI Reference In"=w39, "error in"=w41) -> ("error out"=w40:errorcluster)
  n138 = Release Queue(queue=w31) -> ()  [unwired: 2 in, 3 out]
  n139 = Release Queue(queue=w27) -> ()  [unwired: 2 in, 3 out]
  n140 = flat-sequence {
    tunnel: w40 -> [w343]
    frame #0 {
      n141 = local write "Global Stop"(FALSE ("Global Stop")) -> ()
      "error out" <- w343
    }
  }
